vi "preparetiff.vi"(2 "z":i32, 3 "y":i32, 4 "x":i32, 5 "file path":path) -> (0 "error out":errorcluster, 1 "refnum tif":refnum<file>)   [LabVIEW 2010]
panel:
  out "x*y":i32
  out "IFDend":u32
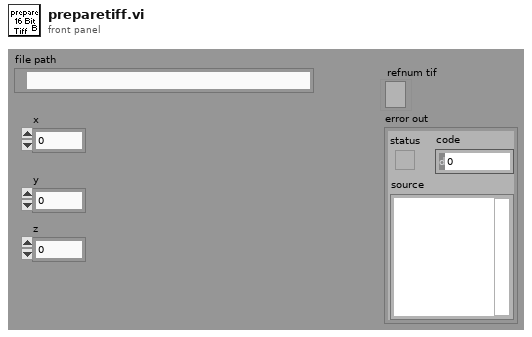
[diagram p1: front panel]
types:
  T1 = enum16{"open", "replace", "create", "open or create", "replace or create", "replace or create with confirmation"}
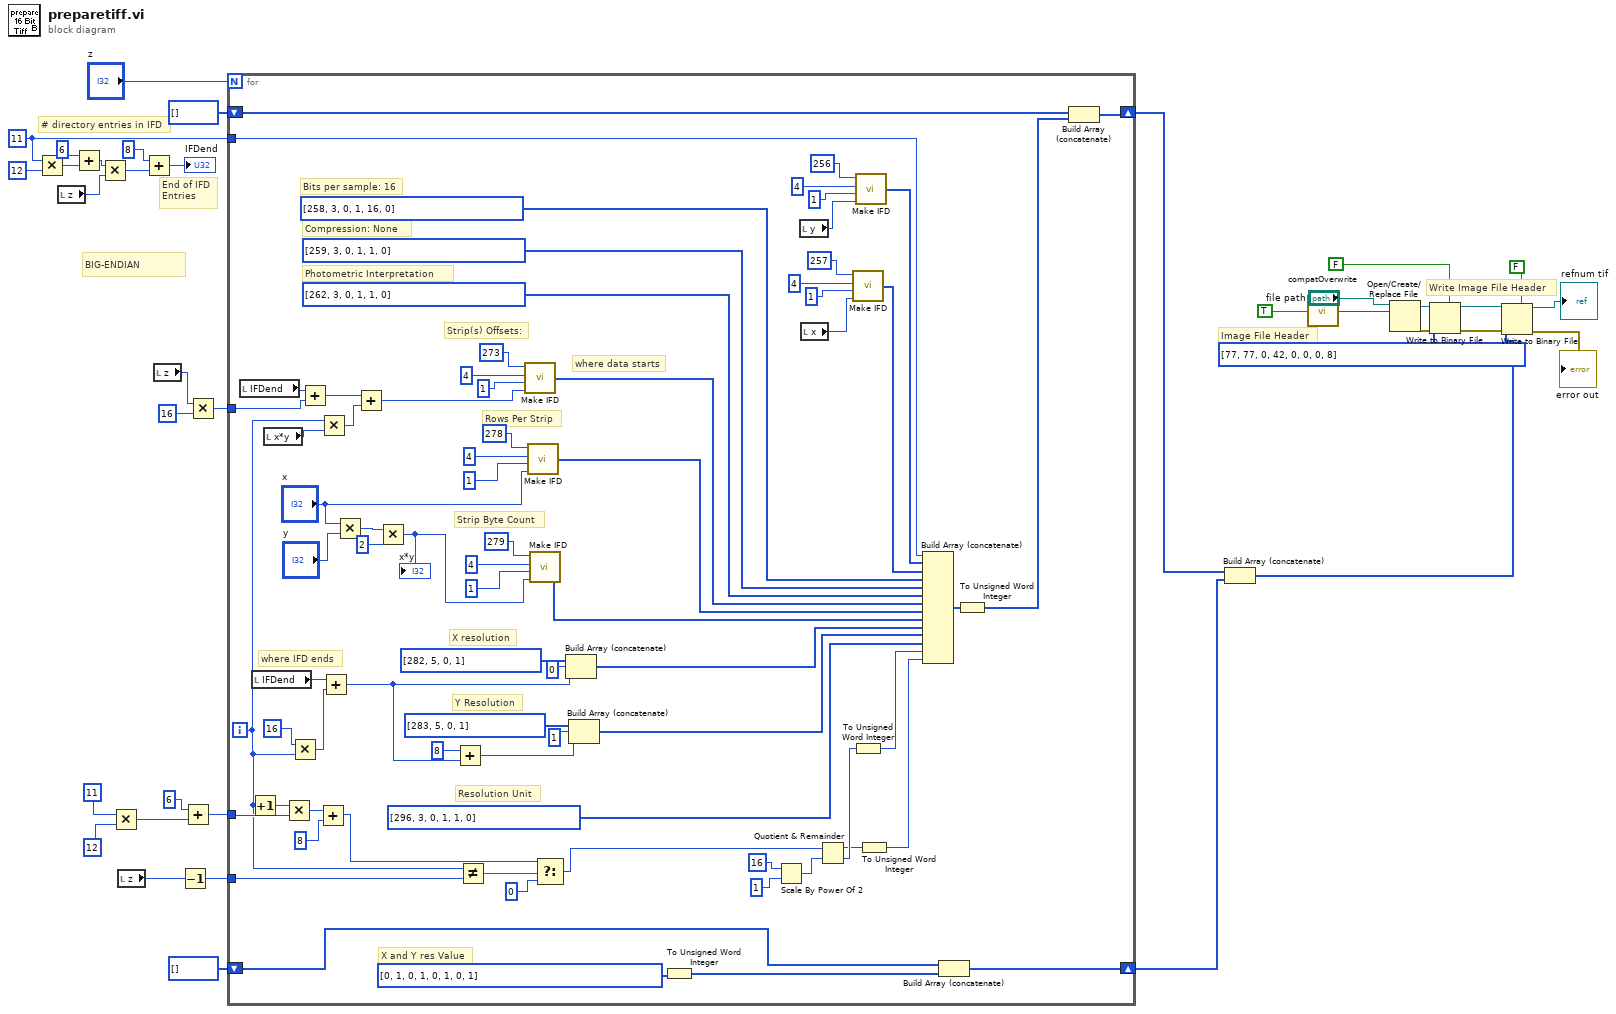
[diagram p0: block diagram]
diagram:
  w29 = u16 11
  # "Image File Header"
  # "Write Image File Header"
  # "End of IFD\nEntries"
  # "# directory entries in IFD"
  # "BIG-ENDIAN"
  n1 = Multiply(x=w29, y=u16 12) -> (x*y=w28:u16)
  n2 = local read "z"() -> (w19:i32)
  n3 = Add(x=u16 6, y=w28) -> (x+y=w22:u16)
  n4 = Multiply(x=w22, y=w19) -> (x*y=w34:i32)
  n5 = Multiply(x=11, y=12) -> (x*y=w24:i32)
  n6 = local read "z"() -> (w17:i32)
  n7 = Add(x=8, y=w34) -> (x+y=→"IFDend":i32)
  n8 = local read "z"() -> (w18:i32)
  n9 = Decrement(x=w17) -> (x-1=w20:i32)
  n10 = Add(x=u16 6, y=w24) -> (x+y=w23:i32)
  n11 = Multiply(x=w18, y=16) -> (x*y=w30:i32)
  n12 = for {
    N: "z" -> [_]
    shift-right: [w66] -> w15
    shift-left: u16[] [] -> [w79]
    shift-right: [w76] -> w14
    shift-left: u16[] [] -> [w75]
    tunnel: w29 -> [w74]
    tunnel: w30 -> [w69]
    tunnel: w23 -> [w63]
    tunnel: w20 -> [w59]
    i -> [w58]
    # "where IFD ends"
    # "where data starts"
    # "X and Y res Value"
    # "Resolution Unit"
    # "Y Resolution"
    # "X resolution"
    # "Bits per sample: 16"
    # "Strip Byte Count"
    # "Rows Per Strip"
    # "Strip(s) Offsets:"
    # "Photometric Interpretation"
    # "Compression: None"
    n13 = local read "IFDend"() -> (w94:u32)
    n14 = Increment(x=w58) -> (x+1=w55:i32)
    n15 = local read "IFDend"() -> (w73:u32)
    n16 = local read "x*y"() -> (w52:i32)
    n17 = Multiply(x=w55, y=w63) -> (x*y=w62:i32)
    n18 = Multiply(x=16, y=w58) -> (x*y=w71:i32)
    n19 = Add(x=w94, y=w69) -> (x+y=w68:u32)
    n20 = Add(x=w62, y=8) -> (x+y=w60:i32)
    n21 = Multiply(x=w58, y=w52) -> (x*y=w67:i32)
    n22 = Add(x=w73, y=w71) -> (x+y=w72:u32)
    n23 = Multiply(x="x", y="y") -> (x*y=w49:i32)
    n24 = Add(x=w68, y=w67) -> (x+y=w65:u32)
    n25 = Multiply(x=w49, y=2) -> (x*y=w48:i32)
    "x*y" <- w48
    n26 = Add(x=u32 8, y=w72) -> (x+y=w64:u32)
    n27 = Not Equal?(x=w58, y=w59) -> (x != y?=w57:bool)
    n28 = call "Make IFD.vi"("Value/Offset"=w65, "Count"=u32 1, "TYPE"=u16 4, "TAG"=u16 273) -> ("IFD entry"=w88:u16[])
    n29 = call "Make IFD.vi"("Value/Offset"="x", "Count"=u32 1, "TYPE"=u16 4, "TAG"=u16 278) -> ("IFD entry"=w87:u16[])
    n30 = call "Make IFD.vi"("Value/Offset"=w48, "Count"=u32 1, "TYPE"=u16 4, "TAG"=u16 279) -> ("IFD entry"=w86:u16[])
    n31 = Select(t=w60, s=w57, f=u16 0) -> (s? t:f=w41:i32)
    n32 = Build Array (concatenate)(u16[] [282, 5, 0, 1], 0, w72) -> (w85:u32[])
    n33 = Build Array (concatenate)(u16[] [283, 5, 0, 1], 1, w64) -> (w84:u32[])
    n34 = To Unsigned Word Integer(number=u16[] [0, 1, 0, 1, 0, 1, 0, 1]) -> (unsigned 16bit integer=w77:u16[])
    n35 = Scale By Power Of 2(n=u32 16, x=u32 1) -> (x*2^n=w44:u32)
    n36 = local read "y"() -> (w53:i32)
    n37 = local read "x"() -> (w54:i32)
    n38 = Quotient & Remainder(x=w41, y=w44) -> (x-y*floor(x/y)=w42:u32, floor(x/y)=w43:u32)
    n39 = call "Make IFD.vi"("Value/Offset"=w54, "Count"=u32 1, "TYPE"=u16 4, "TAG"=u16 257) -> ("IFD entry"=w92:u16[])
    n40 = To Unsigned Word Integer(number=w43) -> (unsigned 16bit integer=w39:u16)
    n41 = call "Make IFD.vi"("Value/Offset"=w53, "Count"=u32 1, "TYPE"=u16 4, "TAG"=u16 256) -> ("IFD entry"=w93:u16[])
    n42 = To Unsigned Word Integer(number=w42) -> (unsigned 16bit integer=w38:u16)
    n43 = Build Array (concatenate)(w74, w93, w92, u16[] [258, 3, 0, 1, 16, 0], u16[] [259, 3, 0, 1, 1, 0], u16[] [262, 3, 0, 1, 1, 0], w88, w87, w86, w85, w84, u16[] [296, 3, 0, 1, 1, 0], w39, w38) -> (w82:u32[])
    n44 = Build Array (concatenate)(w75, w77) -> (w76:u16[])
    n45 = To Unsigned Word Integer(number=w82) -> (unsigned 16bit integer=w40:u16[])
    n46 = Build Array (concatenate)(w79, w40) -> (w66:u16[])
  }
  n47 = Build Array (concatenate)(w15, w14) -> (w13:u16[])
  n48 = call <vilib>:"compatOverwrite.vi"("overwrite (F)"=TRUE) -> ("overwrite?"=w1:T1)
  n49 = Open/Create/Replace File(file path (use dialog)="file path", operation (0:open)=w1) -> (refnum out=w6:refnum<file>, error out=w9:errorcluster)  [unwired: 1 in, 4 out]
  n50 = Write to Binary File(file (use dialog)=w6, data=u8[] [77, 77, 0, 42, 0, 0, 0, 8], error in=w9, 5:FALSE ("prepend array or string size? (T)")) -> (refnum out=w7:refnum<file>, error out=w8:errorcluster)  [unwired: 3 out]
  n51 = Write to Binary File(file (use dialog)=w7, data=w13, error in=w8, 5:FALSE ("prepend array or string size? (T)")) -> (refnum out=→"refnum tif":refnum<file>, error out=→"error out":errorcluster)  [unwired: 3 out]
